vi "WATCH for NOTE.vi"(8 "error in (no error)":errorcluster, 11 "DigitalInputDevRef":T1) -> (0 "error out":errorcluster)   [LabVIEW 2023]
uses:
  <vilib>/Rock Robotics/WPI/DigitalInput/WPI_DigitalInputDevRef.ctl
  <vilib>/Rock Robotics/SystemInterfaces/DIO/FPGA_DIOChannel.ctl
  Global stack names.vi
  <vilib>/Rock Robotics/Network Tables/NT Read Boolean.vi
  <vilib>/Rock Robotics/Network Tables/NT Write Boolean.vi
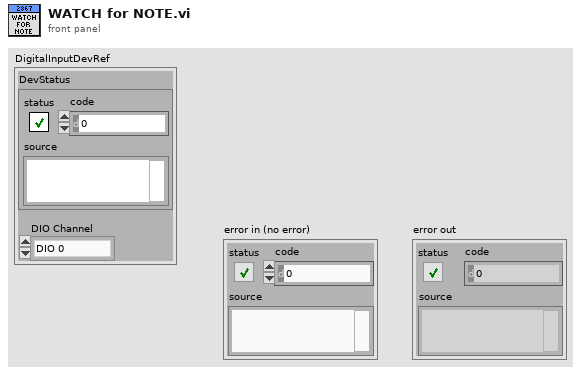
[diagram p1: front panel]
types:
  T1 = typedef "WPI_DigitalInputDevRef.ctl" = cluster{"DevStatus":errorcluster, "DIO Channel":T2}
  T2 = typedef "FPGA_DIOChannel.ctl" = enum8{"DIO 0", "DIO 1", "DIO 2", "DIO 3", "DIO 4", "DIO 5", "DIO 6", "DIO 7", "DIO 8", "DIO 9", "DIO MXP 0", "DIO MXP 1", "DIO MXP 2", "DIO MXP 3", "DIO MXP 4", "DIO MXP 5", "DIO MXP 6", "DIO MXP 7", "DIO MXP 8", "DIO MXP 9", "DIO MXP 10", "DIO MXP 11", "DIO MXP 12", "DIO MXP 13", "DIO MXP 14", "DIO MXP 15", "SPI Port CS1", "SPI Port CS2", "SPI Port CS3", "SPI Port MISO", "SPI Port MOSI", "Invalid"}
  T3 = typedef "ctrl stack - INTAKE SHOOTER.ctl" = cluster{"INTAKE STATE":string, "RUN INTAKE?":string, "RUN REVERSE?":string, "NOTE LOADED?":string, "SHOOTER STATE":string, "SHOOTER FIRE?":string, "SHOOT AMP?":string, "EXTEND FLAP?":string, "LOOKING for NOTE":string, "OVERIDE NOTE CHECK":string}
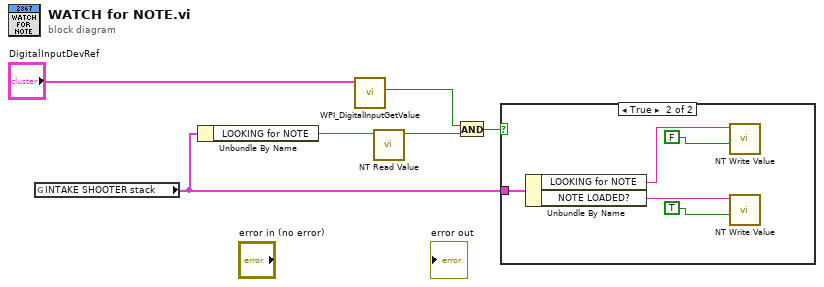
[diagram p0: block diagram]
diagram:
  n1 = global read "Global stack names.vi" "INTAKE SHOOTER stack"() -> (w6:T3)
  n2 = Unbundle By Name(w6) -> ("LOOKING for NOTE"=w4:string)
  n3 = call <vilib>:"WPI_DigitalInputGetValue.vi"("DigitalInputDevRef"="DigitalInputDevRef") -> ("Value"=w1:bool)  [unwired: 8 in, 2 out]
  n4 = call-poly <vilib>:"NT Read Value.vi"("name"=w4) -> ("value"=w3:bool)  [unwired: 8 in, 2 out]
  n5 = And(x=w1, y=w3) -> (x .and. y?=w2:bool)
  n6 = case shown="True" w2 {
    tunnel: w6 -> [_ w7]
    frame False {
    }
    frame True {
      n7 = Unbundle By Name(w7) -> ("LOOKING for NOTE"=w11:string, "NOTE LOADED?"=w10:string)
      n8 = call-poly <vilib>:"NT Write Value.vi"("value"=FALSE, "name"=w11) -> ()  [unwired: 9 in, 1 out]
      n9 = call-poly <vilib>:"NT Write Value.vi"("value"=TRUE, "name"=w10) -> ()  [unwired: 9 in, 1 out]
    }
  }
